vi "DR_Test.vi"() -> ()   [LabVIEW 2015]
panel:
  out "DR Register Value(ms)":dbl=10.0
  out "Period of TIME Data":dbl(graph) caption="Period of TIME Data(New Time Data - Prev Time Data)"
  out "Continuous TIME Data":dbl(graph)
  in  "stop":bool
  in  "DR Rate(ms)":dbl=10.0
  in  "Controller Ip":string="192.168.2.30"
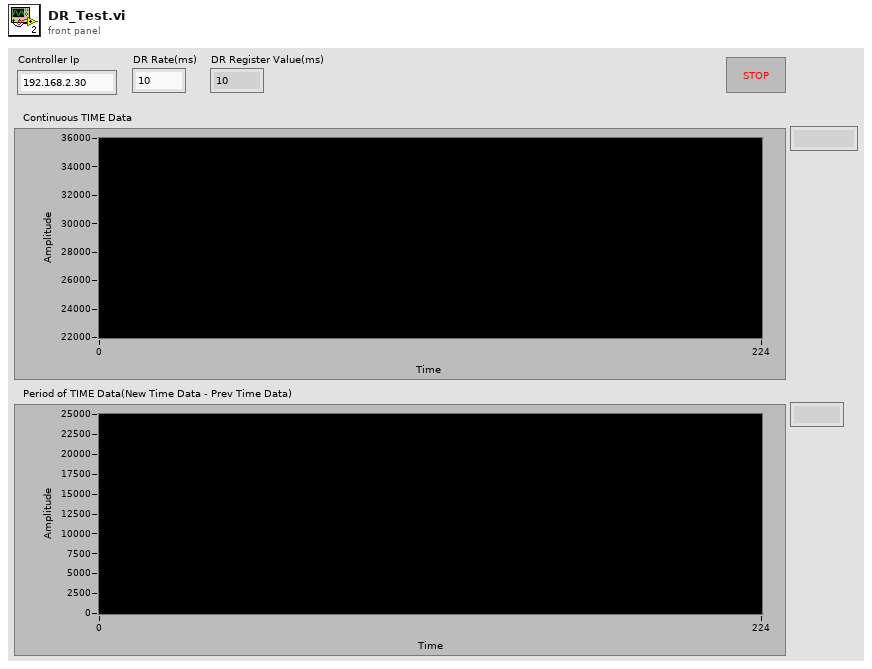
[diagram p1: front panel]
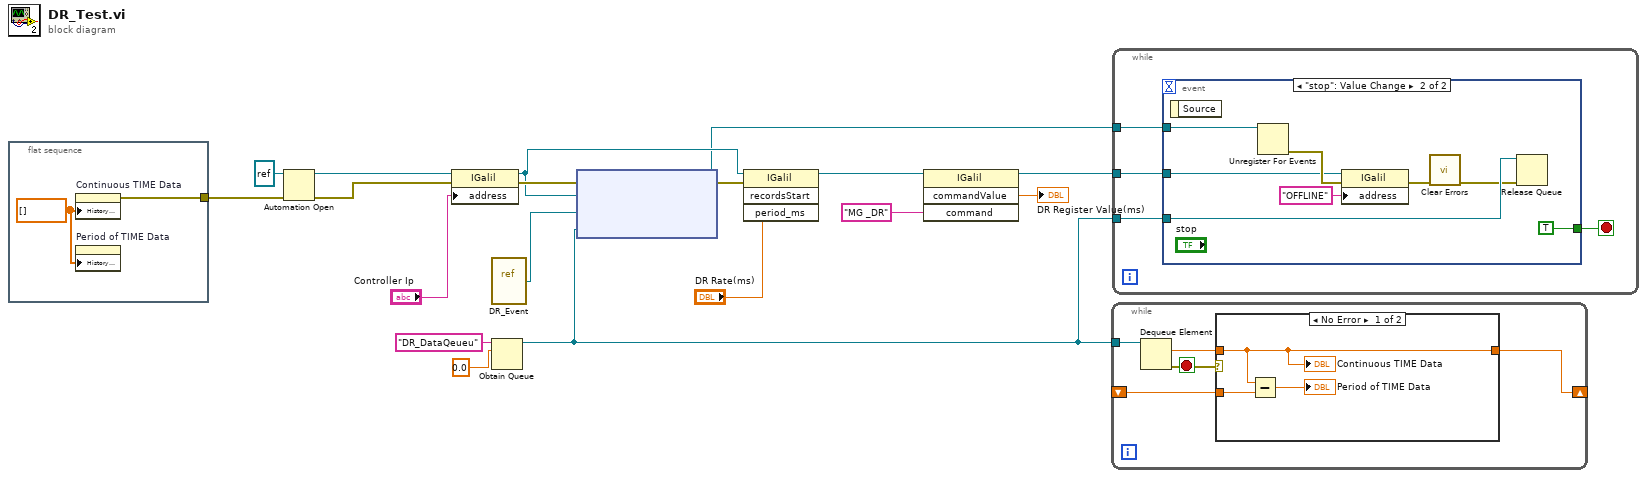
[diagram p0: block diagram]
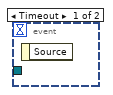
[diagram p3: hidden frame]
diagram:
  n1 = flat-sequence {
    tunnel: [w19] -> w1
    frame #0 {
      w20 = dbl[] [] ("History Data")
      n2 = property on="Continuous TIME Data" class="WFChart (strict)"("History Data"=w20) -> (error out=w19:errorcluster)  [unwired: 2 in, 1 out]
      n3 = property on="Period of TIME Data" class="WFChart (strict)"("History Data"=w20) -> ()  [unwired: 2 in, 2 out]
    }
  }
  n4 = Automation Open(error in (no error)=w1, Automation Refnum=refnum<k7> refnum) -> (Automation Refnum=w16:refnum<k7>, error out=w18:errorcluster)  [unwired: 2 out]
  n5 = property on="Property Node" class="IGalil"(reference=w16, error in=w18, "address"="Controller Ip") -> (reference out=w11:refnum<k7>, error out=w13:errorcluster)
  n6 = vi-ref "DR_Event.vi"() -> ("vi reference"=w14:refnum<vi>)
  n7 = Obtain Queue(name (unnamed)="DR_DataQeueu", element data type=0.0) -> (queue out=w7:refnum<queue>)  [unwired: 3 in, 2 out]
  n8 = node ("Register Event Callback")(w13, w11, w14, w7) -> (w10:refnum<k27>, w12:errorcluster)  [unwired: 1 in]
  n9 = invoke on="Invoke Node" class="IGalil" method="recordsStart"(reference=w11, error in=w12, "period_ms"="DR Rate(ms)") -> (reference out=w5:refnum<k7>)  [unwired: 1 in, 3 out]
  n10 = invoke on="Invoke Node" class="IGalil" method="commandValue"(reference=w5, "command"="MG _DR") -> (reference out=w4:refnum<k7>, "commandValue"=→"DR Register Value(ms)":dbl)  [unwired: 2 in, 2 out]
  n11 = while {
    tunnel: w7 -> [w25]
    shift-right: [w22] -> _
    shift-left: _ -> [w21]
    stop <- w24 stop-if-true
    n12 = Dequeue Element(queue=w25) -> (element=w23:dbl, error out=w24:errorcluster)  [unwired: 2 in, 2 out]
    n13 = case shown="No Error" w24 {
      tunnel: w23 -> [w27 w29]
      tunnel: [w27 w29] -> w22
      tunnel: w21 -> [w28 _]
      frame No Error {
        n14 = Subtract(x=w27, y=w28) -> (x-y=→"Period of TIME Data":dbl)
        "Continuous TIME Data" <- w27
      }
      frame Error {
      }
    }
  }
  n15 = while {
    tunnel: w4 -> [w33]
    tunnel: w10 -> [w32]
    tunnel: w7 -> [w30]
    stop <- w31 stop-if-true
    n16 = event shown="[1] \"stop\": Value Change" {
      selector: _ -> [_ _]
      dyn-events: _ -> [_ _]
      timeout: _ -> [_ _]
      tunnel: w33 -> [_ w37]
      tunnel: w32 -> [_ w38]
      tunnel: [_ TRUE] -> w31
      tunnel: w30 -> [_ w36]
      event Timeout {
        n17 = event-data() -> ()  [unwired: 1 in, 1 out]
      }
      event "stop": Value Change {
        n18 = event-data() -> ()  [unwired: 1 in, 1 out]
        n19 = Unregister For Events(event registration refnum=w38) -> (error out=w40:errorcluster)  [unwired: 1 in]
        n20 = property on="Property Node" class="IGalil"(reference=w37, error in=w40, "address"="OFFLINE") -> (error out=w35:errorcluster)  [unwired: 1 out]
        n21 = call <vilib>:"Clear Errors.vi"("error in (no error)"=w35) -> ("error out"=w34:errorcluster)  [unwired: 5 in, 1 out]
        n22 = Release Queue(queue=w36, error in (no error)=w34) -> ()  [unwired: 1 in, 3 out]
      }
    }
  }
